vi "Escritura en PEM.vi"(0 "Retardo de onda lambda":i32 min=0 max=1000, 1 "Retardo":bool, 2 "VISA resource name":refnum<visa-resource-name>, 3 "Longitud de onda nm":dbl min=0.0 max=19999.9, 4 "error in (no error)":errorcluster) -> (5 "VISA resource name out":refnum<visa-resource-name>, 6 "error out":errorcluster)   [LabVIEW 2018]
panel:
  # "Longitud de onda"
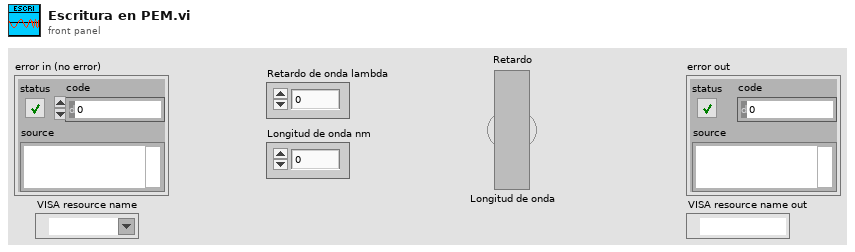
[diagram p1: front panel]
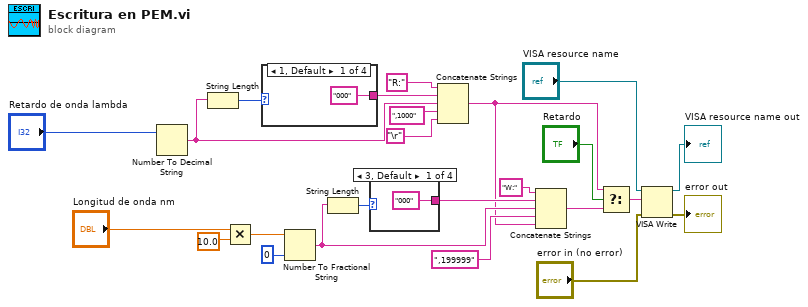
[diagram p0: block diagram]
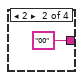
[diagram p2: hidden frame]
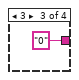
[diagram p3: hidden frame]
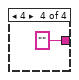
[diagram p4: hidden frame]
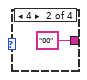
[diagram p5: hidden frame]
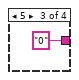
[diagram p6: hidden frame]
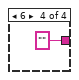
[diagram p7: hidden frame]
diagram:
  n1 = Number To Decimal String(number="Retardo de onda lambda") -> (decimal integer string=w23:string)  [unwired: 1 in]
  n2 = String Length(string=w23) -> (length=w14:i32)
  n3 = Multiply(x="Longitud de onda nm", y=10.0) -> (x*y=w7:dbl)
  n4 = case shown="1, Default" w14 {
    tunnel: ["000" ("string") "00" ("string") "0" ("string") "" ("string")] -> w13
    frame 1, Default {
    }
    frame 2 {
    }
    frame 3 {
    }
    frame 4 {
    }
  }
  n5 = Number To Fractional String(number=w7, precision (6)=i16 0) -> (F-format string=w17:string)  [unwired: 2 in]
  n6 = String Length(string=w17) -> (length=w15:i32)
  n7 = case shown="3, Default" w15 {
    tunnel: ["000" ("string") "00" ("string") "0" ("string") "" ("string")] -> w19
    frame 3, Default {
    }
    frame 4 {
    }
    frame 5 {
    }
    frame 6 {
    }
  }
  n8 = Concatenate Strings("R:" ("string"), w13, w23, ",1000" ("string"), "\r") -> (w5:string)
  n9 = Concatenate Strings("W:" ("string"), w19, w17, ",199999" ("string"), w5) -> (w11:string)
  n10 = Select(t=w5, s="Retardo", f=w11) -> (s? t:f=w10:string)
  n11 = VISA Write(VISA resource name="VISA resource name", write buffer=w10, error in (no error)="error in (no error)") -> (VISA resource name out=→"VISA resource name out":refnum<visa-resource-name>, error out=→"error out":errorcluster)  [unwired: 1 out]
